vi "Table Clear.vi"(8 "Error (In)":errorcluster, 9 "Lvdt":refnum<vi>, 10 "Load":refnum<vi>, 11 "Table (In)":refnum<vi>) -> (0 "Error (Out)":errorcluster, 3 "Table (Out)":refnum<vi>)   [LabVIEW 2020]
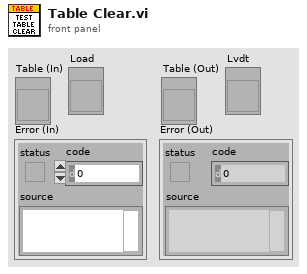
[diagram p1: front panel]
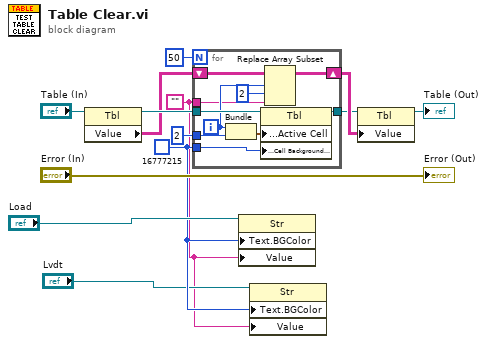
[diagram p0: block diagram]
diagram:
  w1 = ""
  w3 = u32 16777215
  n1 = property class="Tbl"(reference="Table (In)") -> (reference out=w10:refnum<vi>, "Value"=w8:string[][])  [unwired: 1 in, 1 out]
  n2 = for {
    N: 50 -> [_]
    tunnel: w3 -> [w22]
    tunnel: 2 -> [w21]
    tunnel: w10 -> [w20]
    tunnel: [w19] -> w5
    tunnel: w1 -> [w16]
    shift-right: [w14] -> w7
    shift-left: w8 -> [w15]
    i -> [w18]
    n3 = Bundle(w18, w21) -> (w23:cluster{i32, i32})  [unwired: 1 in]
    n4 = property class="Tbl"(reference=w20, "Active Cell:Active Cell"=w23, "Active Cell:Cell Background Color"=w22) -> (reference out=w19:refnum<vi>)  [unwired: 1 in, 1 out]
    n5 = Replace Array Subset(array=w15, new element=w16, index (row)=w18, index (col)=2 ("disabled index (col)")) -> (w14:string[][])
  }
  n6 = property class="Str"(reference="Load", "Text.BGColor"=w3, "Value"=w1) -> ()  [unwired: 1 in, 2 out]
  n7 = property class="Str"(reference="Lvdt", "Text.BGColor"=w3, "Value"=w1) -> ()  [unwired: 1 in, 2 out]
  n8 = property class="Tbl"(reference=w5, "Value"=w7) -> (reference out=→"Table (Out)":refnum<vi>)  [unwired: 1 in, 1 out]
  "Error (Out)" <- "Error (In)"
